vi "BoxSimShoot.vi"() -> ()   [LabVIEW 2023]
uses:
  <vilib>/Rock Robotics/WPI/ThirdParty/JAS_Junk/TrajLib/Enum/DCMOTOR_TYPES_ENUM.ctl
  <vilib>/Rock Robotics/WPI/ThirdParty/JAS_Junk/TrajLib/VI/Util_GetTime_U32.vi
  <vilib>/Rock Robotics/WPI/ThirdParty/JAS_Junk/TrajLib/BatterySim_CalculateLoadedBatteryVoltage.vi
  <vilib>/Rock Robotics/WPI/ThirdParty/JAS_Junk/TrajLib/VI/Util_GetTime_U64.vi
  <vilib>/Rock Robotics/WPI/ThirdParty/JAS_Junk/TrajLib/Trajectory_Library.lvlib
panel:
  out "Shooter Control":T1(graph)
  in  "Auto":bool=TRUE
  out "Velocity_RPM":dbl format="%13.1f"
  out "FeedForward":dbl
  out "AtSetpoint":bool
  in  "Setpoint":dbl
  out "Motor Dmd (CO)":dbl format="%10.3f"
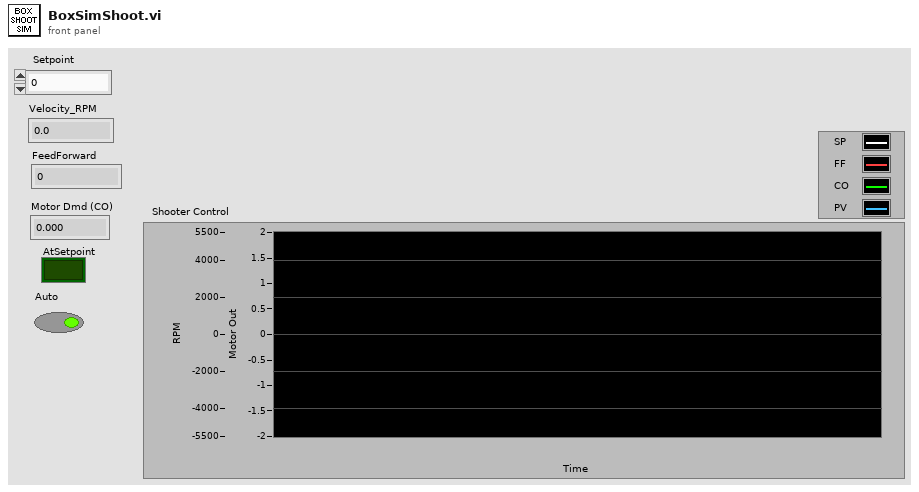
[diagram p1: front panel]
types:
  T1 = cluster{"Setpoint":dbl, "FeedForward":dbl, "CO-ControlOutput":dbl, "Velocity_RPM":dbl}
  T2 = typedef "Trajectory_Library.lvlib/DCMOTOR_TYPES_ENUM.ctl" = enum16{"CIM", "AndyMark 9015", "Andy Mark RS 775 125", "Bag", "BaneBots RS 550", "BaneBots RS 775", "Falcon 500", "Mini CIM", "NEO", "NEO 550", "Romi BuiltIn", "Vex 775 Pro", "Snow Blower AM 2235A", "Bosch Seat AM 3493"}
  T3 = typedef "Trajectory_Library.lvlib/LINEAR_SYSTEM_ID_FLYWHEEL_MODEL.ctl" = cluster{"DCMOTOR_TYPES":T2, "Num Motors":i32, "Gearing":dbl, "MOI kgm2":dbl}
  T4 = typedef "Trajectory_Library.lvlib/FLYWHEEL_SIM_SIMULATION_PARAMS.ctl" = cluster{"Vel Meas Std Dev Rad/Sec":dbl}
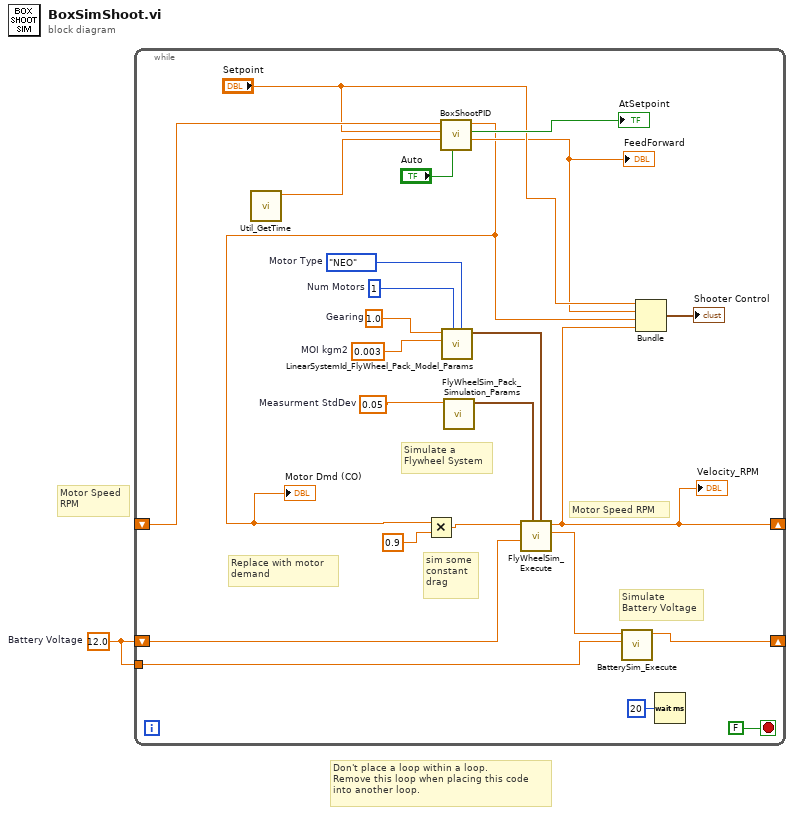
[diagram p0: block diagram]
diagram:
  w1 = 12.0  # Battery Voltage
  # "Don't place a loop within a loop. \nRemove this loop when placing this code\ninto another loop."
  # "Motor Speed\nRPM"
  n1 = while {
    shift-right: [w18] -> _
    shift-left: w1 -> [w17]
    shift-right: [w2] -> _
    shift-left: _ -> [w12]
    tunnel: w1 -> [w13]
    stop <- FALSE stop-if-true
    w15 = 0.05  # Measurment StdDev
    w22 = 1.0  # Gearing
    w23 = 0.003  # MOI kgm2
    w24 = 1  # Num Motors
    w25 = DCMOTOR_TYPES_ENUM."NEO"  # Motor Type
    # "sim some\nconstant\ndrag"
    # "Motor Speed RPM"
    # "Replace with motor \ndemand"
    # "Simulate\nBattery Voltage"
    # "Simulate a \nFlywheel System"
    n2 = call <vilib>:"Util_GetTime.vi"() -> ("FPGA_Time_Seconds"=w11:dbl)  [unwired: 9 in, 2 out]
    n3 = call "BoxShootPID.vi"("Auto"="Auto", "FPGA_Time_Seconds"=w11, "Setpoint"="Setpoint", "Sensor Velocity"=w12) -> ("FeedForward"=w4:dbl, "AtSetpoint"=→"AtSetpoint":bool, "CO-ControlOutput"=w3:dbl)  [unwired: 5 in]
    "Motor Dmd (CO)" <- w3
    "FeedForward" <- w4
    n4 = Multiply(x=w3, y=0.9) -> (x*y=w8:dbl)
    n5 = call <vilib>:"LinearSystemId_FlyWheel_Pack_Model_Params.vi"("DCMOTOR_TYPES"=w25, "Num Motors"=w24, "MOI kgm2"=w23, "Gearing"=w22) -> ("LinearSystem_ID_FlyWheel_Model"=w16:T3)  [unwired: 7 in]
    n6 = call <vilib>:"FlyWheelSim_Pack_Simulation_Params.vi"("Vel Meas StdDev Rad/Sec"=w15) -> ("FlyWheelSim_Simulation_Params"=w14:T4)  [unwired: 10 in]
    n7 = call <vilib>:"FlyWheelSim_Execute.vi"("FlyWheelSim_Model _Params"=w16, "FlyWheelSim_Simulation_Params"=w14, "Battery Volts"=w17, "Motor Dmd"=w8) -> ("Motor Current"=w19:dbl, "Velocity_RPM"=w2:dbl)  [unwired: 4 in, 2 out]
    "Velocity_RPM" <- w2
    n8 = call <vilib>:"BatterySim_Execute.vi"("Nominal Battery Voltage"=w13, "Current"=w19) -> ("Voltage"=w18:dbl)  [unwired: 9 in]
    n9 = Bundle("Setpoint"="Setpoint", "FeedForward"=w4, "CO-ControlOutput"=w3, "Velocity_RPM"=w2) -> (→"Shooter Control":T1)  [unwired: 1 in]
    n10 = Wait (ms)(milliseconds to wait=u32 20) -> ()  [unwired: 1 out]
  }
